vi "Initialize camera.vi"(8 "error in (no error)":errorcluster, 11 "Channel in":refnum<class "Channel.lvclass">) -> (0 "error out":errorcluster, 2 "Initialization":bool, 3 "Channel out":refnum<class "Channel.lvclass">)   [LabVIEW 2018, in "Channel.lvclass"]
doc: "Initialize the camera"
uses:
  Channel.lvclass
  Channel.lvclass/Channel.ctl
  Simulated_CCD_Camera/Simulated Camera.lvclass
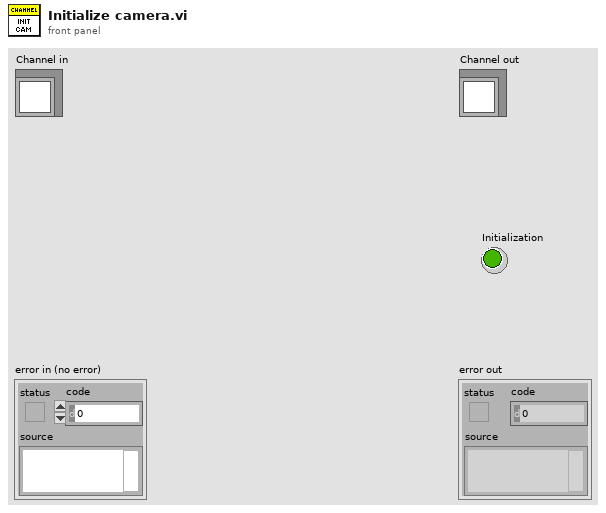
[diagram p1: front panel]
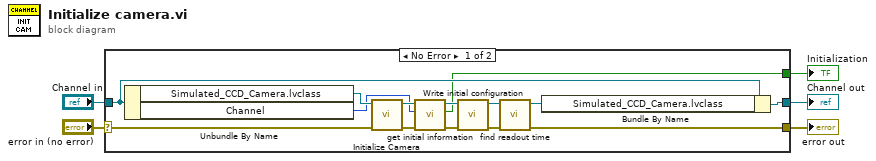
[diagram p0: block diagram]
diagram:
  n1 = case shown="No Error" "error in (no error)" {
    selector: "error in (no error)" -> [w17 w21]
    tunnel: [w8 w21] -> w4
    tunnel: [w16 w20] -> w2
    tunnel: "Channel in" -> [w19 w20]
    tunnel: [w10 _] -> w1
    frame No Error {
      n2 = Unbundle By Name(w19) -> ("Simulated_CCD_Camera.lvclass"=w18:refnum<class "Simulated Camera.lvclass">, "Channel"=w11:u8)
      n3 = call-dynamic "Initialize Camera.vi"("error in (no error)"=w17, "CCDCamera in"=w18) -> ("error out"=w12:errorcluster, "CCDCamera out"=w15:refnum<class "Simulated Camera.lvclass">)  [unwired: 8 in]
      n4 = call-dynamic "get initial information.vi"("error in (no error)"=w12, "channel"=w11, "Simulated_CCD_Camera in"=w15) -> ("error out"=w13:errorcluster, "ccd on/off"=w10:bool, "Simulated_CCD_Camera out"=w14:refnum<class "Simulated Camera.lvclass">)  [unwired: 6 in]
      n5 = call-dynamic "Write initial configuration.vi"("error in (no error)"=w13, "Simulated_CCD_Camera in"=w14) -> ("error out"=w9:errorcluster, "Simulated_CCD_Camera out"=w6:refnum<class "Simulated Camera.lvclass">)  [unwired: 8 in]
      n6 = call "find readout time.vi"("error in (no error)"=w9, "Simulated_CCD_Camera in"=w6) -> ("error out"=w8:errorcluster, "Simulated_CCD_Camera out"=w7:refnum<class "Simulated Camera.lvclass">)  [unwired: 8 in]
      n7 = Bundle By Name(cluster=w19, "Simulated_CCD_Camera.lvclass"=w7) -> (w16:refnum<class "Channel.lvclass">)
    }
    frame Error {
    }
  }
  "error out" <- w4
  "Channel out" <- w2
  "Initialization" <- w1
